vi "process data.vi"(0 "Frequency (Hz)":dbl, 2 "Reference Signal":i32, 5 "sensor input":dbl[][](array[numeric]), 7 "In Signals":dbl[][](array[numeric]), 9 "FFT interval (s)":dbl, 11 "Normalize":bool, 12 "End time (s)":dbl) -> (1 "Fundamental frequency":dbl(slide) scale=0.0..10.0, 3 "FFT":T1, 4 "peaks":dbl[][](array[numeric]), 6 "Magnitude of time data":cluster{dbl[], dbl[]}, 8 "x',y',z'":T2, 10 "Signals":dbl[][](array[numeric]), 14 "Filtered signal":dbl[](graph), 15 "max amplitude":dbl(slide) scale=0.0..6.0)   [LabVIEW 2009]
panel:
  out "Frequency (Hz) 2":dbl
  out "Matched signal":dynamicdata(graph)
  out "max correlation Secondary":dbl(slide) scale=0.0..1.0
  out "max correlation Primary":dbl(slide) scale=0.0..1.0
  out "peak big":dbl[](array[numeric])
  out "peak med":dbl[](array[numeric])
  out "peak small":dbl[](array[numeric])
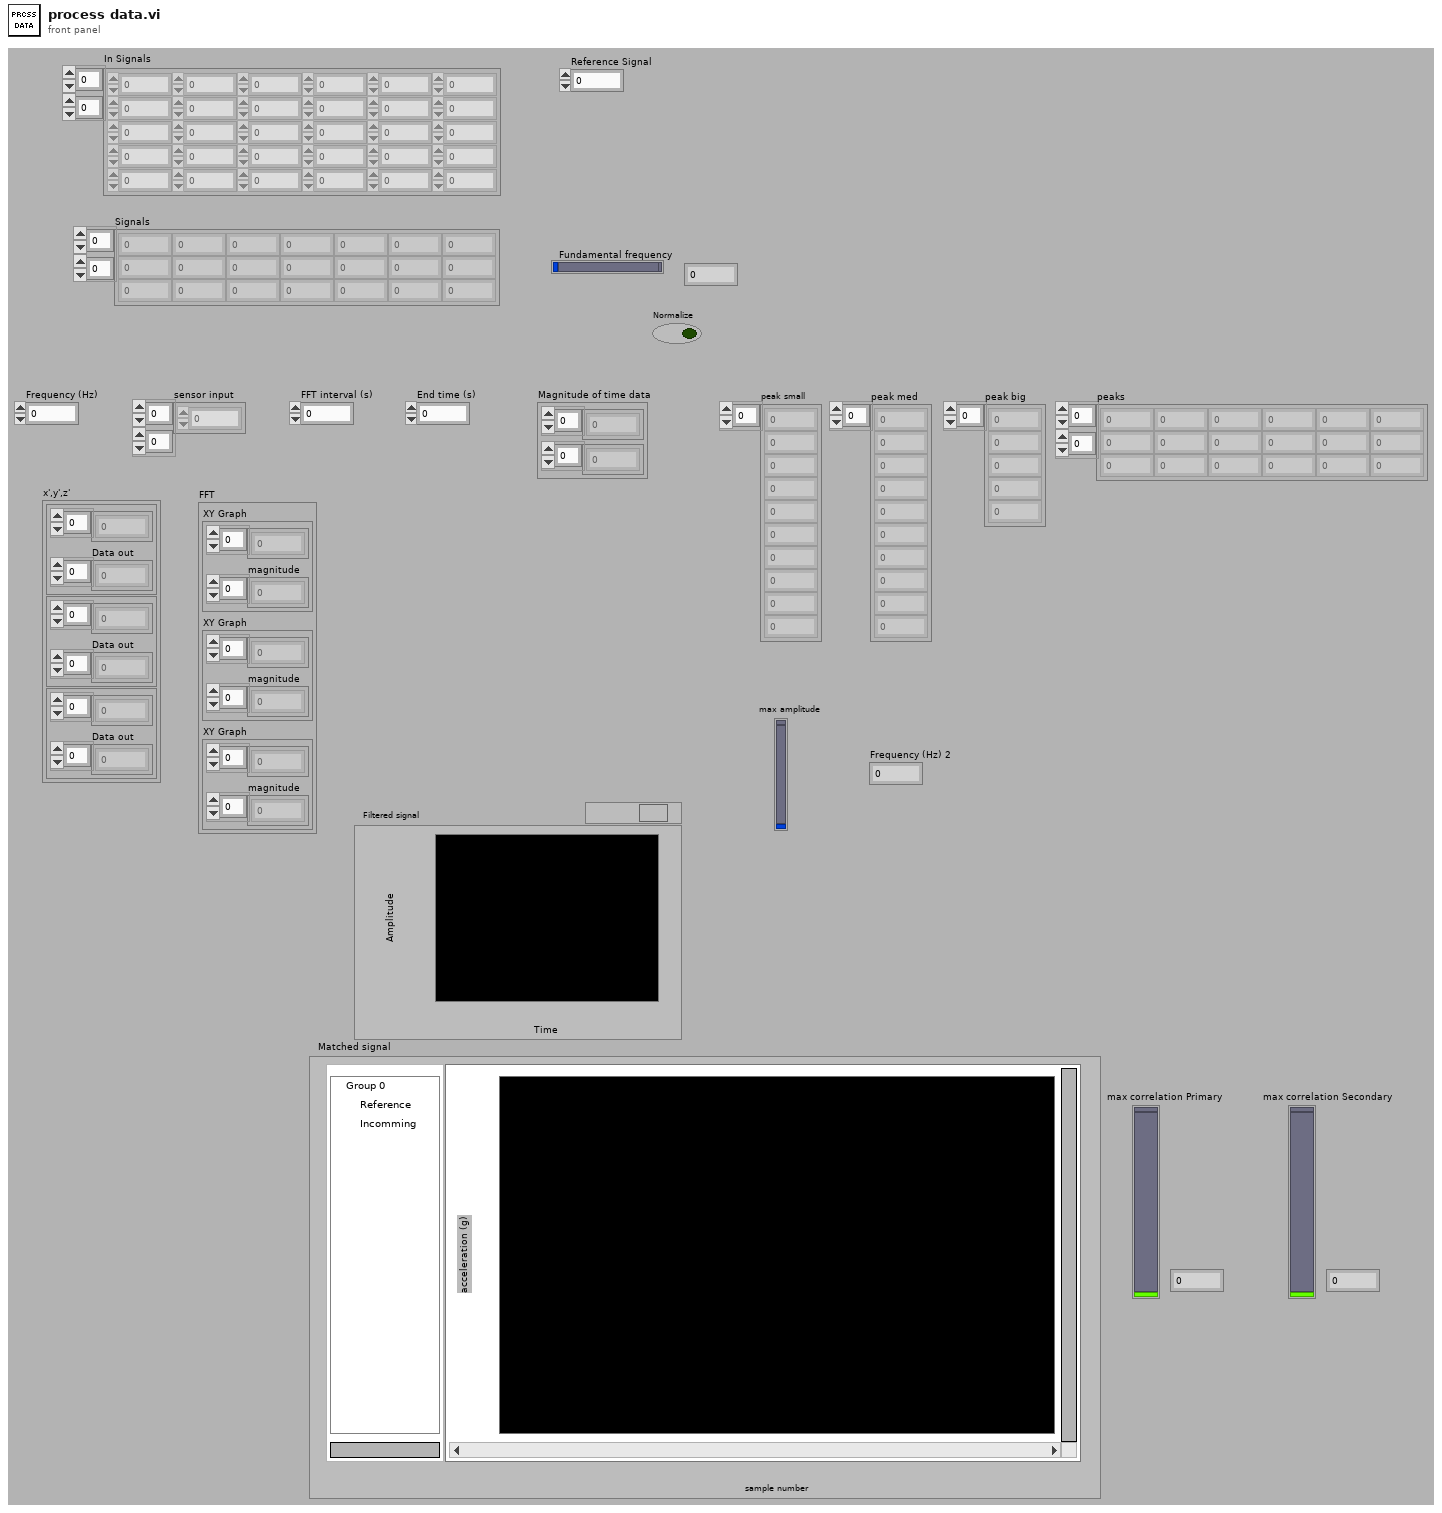
[diagram p1: front panel]
types:
  T1 = cluster{"XY Graph":cluster{dbl[], "magnitude":dbl[]}, "XY Graph":cluster{dbl[], "magnitude":dbl[]}, "XY Graph":cluster{dbl[], "magnitude":dbl[]}}
  T2 = cluster{cluster{dbl[], "Data out":dbl[]}, cluster{dbl[], "Data out":dbl[]}, cluster{dbl[], "Data out":dbl[]}}
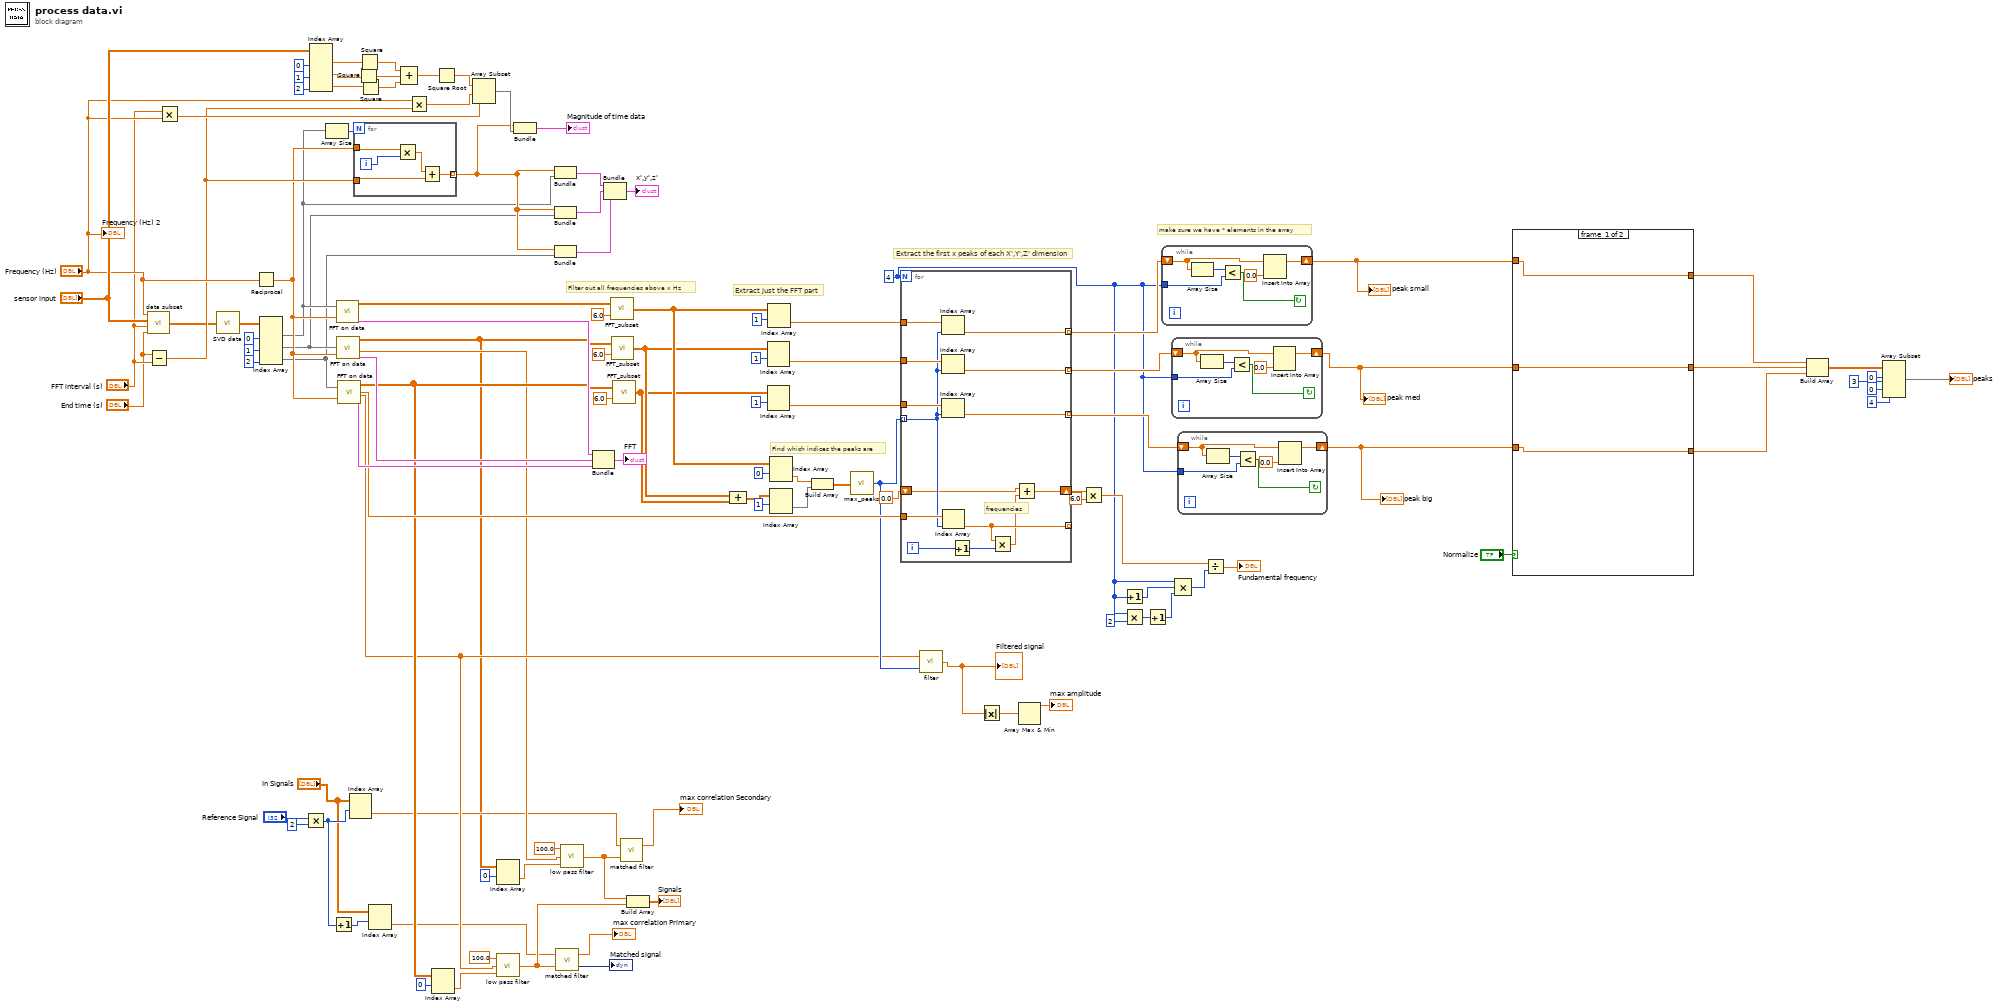
[diagram p0: block diagram]
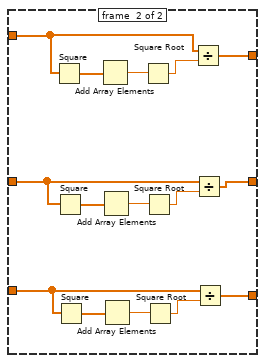
[diagram p2: hidden frame]
diagram:
  w36 = 4
  # "make sure we have * elements in the array"
  # "Extract the first x peaks of each X',Y',Z' dimension"
  # "Find which indices the peaks are"
  # "Filter out all frequencies above x Hz"
  # "Extract just the FFT part"
  n1 = call "data subset.vi"("End time (s)"="End time (s)", "FFT interval (s)"="FFT interval (s)", "sensor"="sensor input", "Frequency (Hz)"="Frequency (Hz)") -> ("sensor subset"=w1:dbl[][])
  n2 = Subtract(x="End time (s)", y="FFT interval (s)") -> (x-y=w106:dbl)
  n3 = Multiply(x="FFT interval (s)", y="Frequency (Hz)") -> (x*y=w111:dbl)
  n4 = call "SVD data.vi"("Data"=w1) -> ("Data out"=w84:dbl[][])
  n5 = Reciprocal(x="Frequency (Hz)") -> (1/x=w80:dbl)
  n6 = Index Array(array=w84, index (col) #1=0 ("disabled index (col)"), index (col) #2=1 ("index (col)"), index (col) #3=2 ("index (col)")) -> (element #1=w52:dbl[], element #2=w51:dbl[], element #3=w2:dbl[])  [unwired: 3 in]
  n7 = Multiply(x="Reference Signal", y=2) -> (x*y=w8:i32)
  n8 = Index Array(array="sensor input", index (col) #1=0 ("disabled index (col)"), index (col) #2=1 ("index (col)"), index (col) #3=2 ("index (col)")) -> (element #1=w97:dbl[], element #2=w96:dbl[], element #3=w98:dbl[])  [unwired: 3 in]
  n9 = Array Size(array=w52) -> (size(s)=w88:i32)
  n10 = Increment(x=w8) -> (x+1=w6:i32)
  n11 = call "FFT on data.vi"("dt"=w80, "Data"=w52) -> ("XY Graph"=w79:cluster{dbl[], "magnitude":dbl[]}, "output"=w26:dbl[][])  [unwired: 3 out]
  n12 = call "FFT on data.vi"("dt"=w80, "Data"=w51) -> ("XY Graph"=w78:cluster{dbl[], "magnitude":dbl[]}, "FFT {X}"=w15:cdb[], "output"=w3:dbl[][])  [unwired: 2 out]
  n13 = call "FFT on data.vi"("dt"=w80, "Data"=w2) -> ("XY Graph"=w103:cluster{dbl[], "magnitude":dbl[]}, "FFT {X}"=w20:cdb[], "output"=w21:dbl[][], "frequency (Hz)"=w43:dbl[])  [unwired: 1 out]
  n14 = Index Array(array="In Signals", index (row)=w8) -> (element=w9:dbl[])  [unwired: 1 in]
  n15 = for {
    N: w88 -> [_]
    tunnel: w80 -> [w118]
    tunnel: w106 -> [w116]
    tunnel: [w114] -> w104 mode=indexing
    i -> [w117]
    n16 = Multiply(x=w118, y=w117) -> (x*y=w115:dbl)
    n17 = Add(x=w115, y=w116) -> (x+y=w114:dbl)
  }
  n18 = Square(x=w96) -> (x^2=w100:dbl[])
  n19 = Square(x=w97) -> (x^2=w99:dbl[])
  n20 = Square(x=w98) -> (x^2=w101:dbl[])
  n21 = Index Array(array="In Signals", index (row)=w6) -> (element=w5:dbl[])  [unwired: 1 in]
  n22 = Compound Arithmetic op=ADD(w99, w100, w101) -> (w102:dbl[])
  n23 = Multiply(x="Frequency (Hz)", y=w106) -> (x*y=w107:dbl)
  n24 = Index Array(array=w21, index (row)=0 ("disabled index (col)")) -> (element=w25:dbl[])  [unwired: 1 in]
  n25 = Square Root(x=w102) -> (sqrt(x)=w108:dbl[])
  n26 = Array Subset(array=w108, index=w107, length=w111) -> (w109:dbl[])
  n27 = Index Array(array=w3, index (row)=0 ("disabled index (col)")) -> (element=w19:dbl[])  [unwired: 1 in]
  n28 = call "low pass filter.vi"("Input frequencies"=w25, "input FFT"=w20, "cut off frequency"=100.0) -> ("Output Time Domain"=w13:dbl[])
  n29 = Bundle(w104, w109) -> (→"Magnitude of time data":cluster{dbl[], dbl[]})  [unwired: 1 in]
  n30 = Bundle(w104, "Data out"=w52) -> (w90:cluster{dbl[], "Data out":dbl[]})  [unwired: 1 in]
  n31 = Bundle(w104, "Data out"=w51) -> (w91:cluster{dbl[], "Data out":dbl[]})  [unwired: 1 in]
  n32 = Bundle(w104, "Data out"=w2) -> (w92:cluster{dbl[], "Data out":dbl[]})  [unwired: 1 in]
  n33 = call "matched filter.vi"("incoming signal"=w13, "reference signal"=w5) -> ("Matched signal"=→"Matched signal":dynamicdata, "max correlation"=→"max correlation Primary":dbl)
  n34 = call "low pass filter.vi"("Input frequencies"=w19, "input FFT"=w15, "cut off frequency"=100.0) -> ("Output Time Domain"=w14:dbl[])
  n35 = Bundle("XY Graph"=w79, "XY Graph"=w78, "XY Graph"=w103) -> (→"FFT":T1)  [unwired: 1 in]
  n36 = Bundle(w90, w91, w92) -> (→"x',y',z'":T2)  [unwired: 1 in]
  n37 = call "FFT_subset.vi"("Hz"=6.0, "input"=w26) -> ("subarray"=w72:dbl[][])
  n38 = call "FFT_subset.vi"("Hz"=6.0, "input"=w3) -> ("subarray"=w69:dbl[][])
  n39 = call "FFT_subset.vi"("Hz"=6.0, "input"=w21) -> ("subarray"=w67:dbl[][])
  n40 = call "matched filter.vi"("incoming signal"=w14, "reference signal"=w9) -> ("max correlation"=→"max correlation Secondary":dbl)  [unwired: 1 out]
  n41 = Build Array(w14, w13) -> (→"Signals":dbl[][])
  n42 = Compound Arithmetic op=ADD(w69, w67) -> (w77:dbl[][])
  n43 = Index Array(array=w69, index (row)=1) -> (element=w65:dbl[])  [unwired: 1 in]
  n44 = Index Array(array=w67, index (row)=1) -> (element=w64:dbl[])  [unwired: 1 in]
  n45 = Index Array(array=w72, index (row)=1) -> (element=w70:dbl[])  [unwired: 1 in]
  n46 = Index Array(array=w72, index (row)=0) -> (element=w75:dbl[])  [unwired: 1 in]
  n47 = Index Array(array=w77, index (row)=1) -> (element=w74:dbl[])  [unwired: 1 in]
  n48 = Build Array(w75, w74) -> (w73:dbl[][])
  n49 = call "max_peaks.vi"("FFT in"=w73) -> ("peak indices"=w31:i32[])
  n50 = for {
    N: w36 -> [_]
    tunnel: w31 -> [w125] mode=indexing
    tunnel: w70 -> [w132]
    tunnel: w65 -> [w131]
    tunnel: w64 -> [w130]
    tunnel: [w129] -> w61 mode=indexing
    tunnel: [w128] -> w60 mode=indexing
    tunnel: [w127] -> w59 mode=indexing
    tunnel: w43 -> [w126]
    tunnel: [w122] -> _ mode=indexing
    shift-right: [w119] -> w41
    shift-left: 0.0 -> [w120]
    i -> [w124]
    # "frequencies"
    n51 = Index Array(array=w132, index=w125) -> (element=w129:dbl)
    n52 = Index Array(array=w131, index=w125) -> (element=w128:dbl)
    n53 = Index Array(array=w130, index=w125) -> (element=w127:dbl)
    n54 = Index Array(array=w126, index=w125) -> (element=w122:dbl)
    n55 = Increment(x=w124) -> (x+1=w123:i32)
    n56 = Multiply(x=w122, y=w123) -> (x*y=w121:dbl)
    n57 = Add(x=w120, y=w121) -> (x+y=w119:dbl)
  }
  n58 = call "filter.vi"("peak indices"=w31, "FFT{x}"=w20) -> ("X"=w30:dbl[])
  "Filtered signal" <- w30
  n59 = Absolute Value(x=w30) -> (abs(x)=w29:dbl[])
  n60 = Array Max & Min(array=w29) -> (max value=→"max amplitude":dbl)  [unwired: 3 out]
  n61 = Multiply(x=w41, y=6.0) -> (x*y=w39:dbl)
  n62 = Increment(x=w36) -> (x+1=w35:i32)
  n63 = Multiply(x=w36, y=2) -> (x*y=w37:i32)
  n64 = Increment(x=w37) -> (x+1=w34:i32)
  n65 = while {
    tunnel: w36 -> [w137]
    shift-right: [w133] -> w44
    shift-left: w61 -> [w135]
    stop <- w136 continue-if-true
    n66 = Array Size(array=w135) -> (size(s)=w138:i32)
    n67 = Less?(x=w138, y=w137) -> (x < y?=w136:bool)
    n68 = Insert Into Array(array=w135, new element=0.0 ("new element/subarray")) -> (w133:dbl[])  [unwired: 1 in]
  }
  "peak small" <- w44
  n69 = while {
    tunnel: w36 -> [w143]
    shift-right: [w139] -> w48
    shift-left: w60 -> [w141]
    stop <- w142 continue-if-true
    n70 = Array Size(array=w141) -> (size(s)=w144:i32)
    n71 = Less?(x=w144, y=w143) -> (x < y?=w142:bool)
    n72 = Insert Into Array(array=w141, new element=0.0 ("new element/subarray")) -> (w139:dbl[])  [unwired: 1 in]
  }
  "peak med" <- w48
  n73 = Compound Arithmetic op=MULTIPLY(w36, w35, w34) -> (w33:i32)
  n74 = while {
    tunnel: w36 -> [w149]
    shift-right: [w145] -> w50
    shift-left: w59 -> [w147]
    stop <- w148 continue-if-true
    n75 = Array Size(array=w147) -> (size(s)=w150:i32)
    n76 = Less?(x=w150, y=w149) -> (x < y?=w148:bool)
    n77 = Insert Into Array(array=w147, new element=0.0 ("new element/subarray")) -> (w145:dbl[])  [unwired: 1 in]
  }
  "peak big" <- w50
  n78 = Divide(x=w39, y=w33) -> (x/y=→"Fundamental frequency":dbl)
  n79 = case shown="False" "Normalize" {
    tunnel: w50 -> [w151 w165]
    tunnel: [w151 w164] -> w49
    tunnel: w48 -> [w152 w157]
    tunnel: [w152 w156] -> w47
    tunnel: w44 -> [w153 w155]
    tunnel: [w153 w154] -> w46
    frame #0 {
    }
    frame #1 {
      n80 = Square(x=w155) -> (x^2=w161:dbl[])
      n81 = Square(x=w157) -> (x^2=w163:dbl[])
      n82 = Square(x=w165) -> (x^2=w168:dbl[])
      n83 = Add Array Elements(numeric array=w161) -> (sum=w160:dbl)
      n84 = Add Array Elements(numeric array=w163) -> (sum=w162:dbl)
      n85 = Add Array Elements(numeric array=w168) -> (sum=w167:dbl)
      n86 = Square Root(x=w160) -> (sqrt(x)=w159:dbl)
      n87 = Square Root(x=w162) -> (sqrt(x)=w158:dbl)
      n88 = Square Root(x=w167) -> (sqrt(x)=w166:dbl)
      n89 = Divide(x=w155, y=w159) -> (x/y=w154:dbl[])
      n90 = Divide(x=w157, y=w158) -> (x/y=w156:dbl[])
      n91 = Divide(x=w165, y=w166) -> (x/y=w164:dbl[])
    }
  }
  n92 = Build Array(w46, w47, w49) -> (w54:dbl[][])
  n93 = Array Subset(array=w54, index (row)=0 ("index"), length (row)=3 ("length"), index (col)=0 ("index"), length (col)=4 ("length")) -> (→"peaks":dbl[][])
  "Frequency (Hz) 2" <- "Frequency (Hz)"
